vi "4_10.vi"() -> ()   [LabVIEW 2020]
panel:
  in  "Extract":string
  out "Output":string[](array[string])
  in  "Word":string
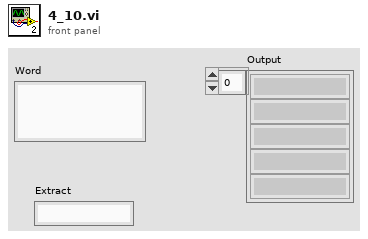
[diagram p1: front panel]
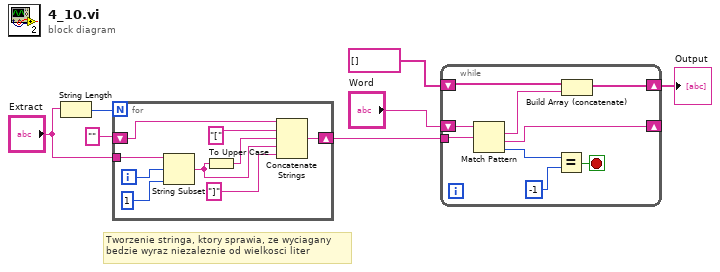
[diagram p0: block diagram]
diagram:
  # "Tworzenie stringa, ktory sprawia, ze wyciagany\nbedzie wyraz niezaleznie od wielkosci liter"
  n1 = String Length(string="Extract") -> (length=w2:i32)
  n2 = for {
    N: w2 -> [_]
    tunnel: "Extract" -> [w16]
    shift-right: [w12] -> w3
    shift-left: "" -> [w11]
    i -> [w13]
    n3 = String Subset(string=w16, offset (0)=w13, length (rest)=1 ("length (rest)")) -> (substring=w9:string)
    n4 = To Upper Case(1:w9) -> (0:w8:string)
    n5 = Concatenate Strings(w11, "[", w8, w9, "]") -> (w12:string)
  }
  n6 = while {
    shift-right: [w21] -> _
    shift-left: "Word" -> [w25]
    shift-right: [w19] -> w6
    shift-left: string[] [] -> [w20]
    tunnel: w3 -> [w17]
    stop <- w22 stop-if-true
    n7 = Match Pattern(string=w25, regular expression=w17) -> (match substring=w18:string, after substring=w21:string, offset past match=w24:i32)  [unwired: 1 in, 1 out]
    n8 = Equal?(x=w24, y=-1) -> (x = y?=w22:bool)
    n9 = Build Array (concatenate)(w20, w18) -> (w19:string[])
  }
  "Output" <- w6
